vi "fpgaDMA Transfer Process.vi"(6 "DMA Write Timed Out?":bool, 7 "Clock Domain":refnum<k21>="40 MHz Onboard Clock", 10 "Local":refnum<k21>, 11 "DMA":refnum<k21>) -> ()   [LabVIEW 2012]
uses:
  <vilib>/Platform/TimedLoop/XDataNode/timing_clust.ctl
  <vilib>/Platform/TimedLoop/XDataNode/nitl_modes.ctl
  <vilib>/Platform/TimedLoop/XDataNode/wakeup.ctl
  <vilib>/rvi/Emulation/niFpgaSctlEmulationRegisterWithScheduler.vi
  <vilib>/rvi/DataTransferAndStorage/Container/Common/niFpgaContainerExecOnDevCompGetState.vi
  <vilib>/rvi/DataTransferAndStorage/Container/Common/niFpgaContainerGetUniqueNameForEmu.vi
  <vilib>/rvi/FIFO/Fifo_Resource/nirvififoEmulationSetSize.vi
  <vilib>/rvi/Emulation/niFpgaSctlEmulationFifoFullMgr.vi
  <vilib>/rvi/errors/niFpgaSetErrorForExecOnDevCompSimple.vi
  <vilib>/rvi/eio/common/nirviEmuReportErrorAndStop.vi
  <vilib>/rvi/interface/RandomDataEmulation/nirviRandomDataFPGAFIFO.vi
  <vilib>/rvi/interface/RandomDataEmulation/niFpgaRandomDataHandleErrors.vi
  <vilib>/rvi/Emulation/niFpgaSctlEmulationResourceMgr.vi
  <vilib>/rvi/Emulation/niFpgaSctlEmulationScheduler.vi
  <vilib>/Platform/TimedLoop/XDataNode/XDataNode.xnode
  <vilib>/rvi/DataTransferAndStorage/Container/XNode/niFpgaContainer.xnode
  <vilib>/rvi/FIFO/Fifo_Resource/niFpgaFifoEmulationRefIn.vi
  <vilib>/Platform/TimedLoop/XDataNode/XDNodeRunTimeDep.lvlib
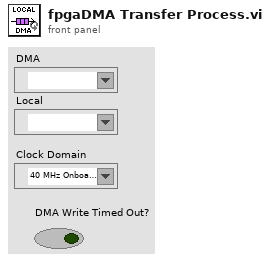
[diagram p1: front panel]
types:
  T1 = typedef "XDNodeRunTimeDep.lvlib/timing_clust.ctl" = cluster{"Expected End [f-1]":u64, "Actual End [f-1]":u64, "Finished Late? [f-1]":bool, "Expected End [i-1]":u64, "Actual End [i-1]":u64, "Finished Late? [i-1]":bool, "Expected Start [i]":u64, "Actual Start [i]":u64, "Expected Start [f]":u64, "Actual Start [f]":u64, "Source Name":string, "Structure Name":string, "Period":i64, "Deadline":i64, "Offset":i64, "Start":i64, "Priority":i32, "Timeout":i32, "Mode":T2, "Wakeup Reason":T3, "Error":errorcluster, "Source Type":string, "Secondary Source Type":string, "Global End Time":u64, "Global Start Time":u64, "Frame Duration":u64, "Iteration Duration":u64, "Assigned CPU":i32, "I/O Scan Engine Mode":u32}
  T2 = typedef "XDNodeRunTimeDep.lvlib/nitl_modes.ctl" = enum32{"No Change", "Process missed periods, maintain original phase", "Discard missed periods, maintain original phase", "Process missed periods, ignore original phase", "Discard missed periods, ignore original phase"}
  T3 = typedef "XDNodeRunTimeDep.lvlib/wakeup.ctl" = enum32{"Normal", "Aborted", "Asynchronous wakeup", "Timing source error", "Timed loop error", "Timeout"}
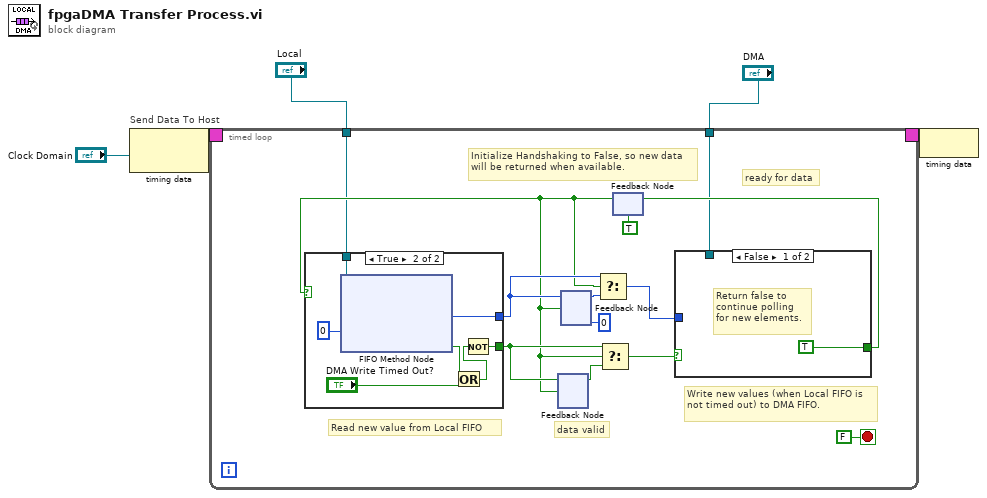
[diagram p0: block diagram]
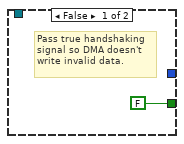
[diagram p2: hidden frame]
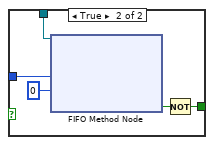
[diagram p3: hidden frame]
diagram:
  n1 = node-c288("Clock Domain") -> (w5:T1)
  n2 = timed-loop "Send Data To Host" {
    timing: w5 -> [_]
    timing-out: [_] -> w4
    tunnel: "DMA" -> [w7]
    tunnel: "Local" -> [w6]
    stop <- FALSE stop-if-true
    # "Read new value from Local FIFO"
    # "ready for data"
    # "data valid"
    # "Initialize Handshaking to False, so new data will be returned when available."
    # "Write new values (when Local FIFO is not timed out) to DMA FIFO."
    n3 = feedback #1() -> (w10:bool)  [unwired: 1 in]
    n4 = feedback #2(i16 0 ("Element")) -> (w14:i16)
    n5 = feedback #3(TRUE ("Timed Out?")) -> (w9:bool)
    n6 = case shown="True" w9 {
      tunnel: [FALSE ("Timed Out?") w26] -> w11
      tunnel: [_ w24] -> w13
      tunnel: w6 -> [_ w23]
      frame False {
        # "Pass true handshaking\nsignal so DMA doesn't\nwrite invalid data."
      }
      frame True {
        n7 = xnode ("FIFO Method Node")("Timeout"=0, "FIFO In"=w23) -> ("Element"=w24:i16, "Timed Out?"=w22:bool)  [unwired: 1 out]
        n8 = Or(x=w22, y="DMA Write Timed Out?") -> (x .or. y?=w20:bool)
        n9 = Not(x=w20) -> (.not. x?=w26:bool)
      }
    }
    n10 = feedback-in #1(w11, w9) -> ()
    n11 = feedback-in #2(w13, w9) -> ()
    n12 = Select(t=w13, s=w9, f=w14) -> (s? t:f=w15:i16)
    n13 = Select(t=w11, s=w9, f=w10) -> (s? t:f=w8:bool)
    n14 = case shown="False" w8 {
      tunnel: [TRUE ("Timed Out?") w32] -> w16
      tunnel: w15 -> [_ w31]
      tunnel: w7 -> [_ w28]
      frame False {
        # "Return false to \ncontinue polling\nfor new elements."
      }
      frame True {
        n15 = xnode ("FIFO Method Node")("Element"=w31, "Timeout"=0, "FIFO In"=w28) -> ("Timed Out?"=w29:bool)  [unwired: 1 out]
        n16 = Not(x=w29) -> (.not. x?=w32:bool)
      }
    }
    n17 = feedback-in #3(w16) -> ()
  }
  n18 = node-c288(w4) -> ()
